vi "poly_set_xwav_xdim.vi"(1 "x dim (x)":string="au", 3 "xwave in":T1={"attributes"=variant, "X"={"start"=0.0, "delta"=0.0, "units"="index", "dim"="au"}, "Y"={"data"=[], "units"="au"}}) -> (0 "xwave out":T1={"attributes"=variant, "X"={"start"=0.0, "delta"=0.0, "units"="index", "dim"="au"}, "Y"={"data"=[], "units"="au"}})   [LabVIEW 2015, in "_xwav_polys.lvlib"]
uses:
  _xwav_polys.lvlib
  xwav.ctl
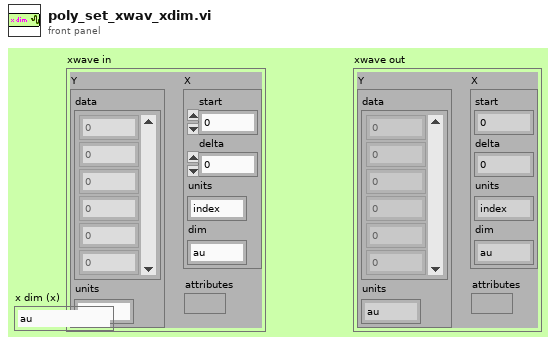
[diagram p1: front panel]
types:
  T1 = typedef "xwav.ctl" = cluster{"attributes":variant, "X":cluster{"start":dbl, "delta":dbl, "units":string, "dim":string}, "Y":cluster{"data":dbl[], "units":string}}
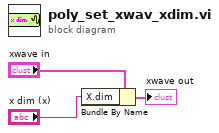
[diagram p0: block diagram]
diagram:
  n1 = Bundle By Name(cluster="xwave in", "X.dim"="x dim (x)") -> (→"xwave out":T1)
